vi "Calculate Tau Error.vi"(1 "tau":dbl, 2 "Dt":dbl, 3 "X":dbl[](array[numeric]), 4 "A":dbl, 8 "B":dbl) -> (7 "e_tau":dbl)   [LabVIEW 2019, in "Math Utilities.lvlib"]
doc: "Calculate the error in the fitted coefficient tau according to Halmer et al. [2004, Rev. Sci. Instr.]. The error will be the standard deviation of the fit (with N-3 degrees of freedom) multiplied by the sum of the square of the derivative of the exponential equation at each point in time."
uses:
  Math Utilities.lvlib
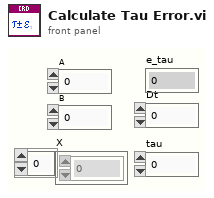
[diagram p1: front panel]
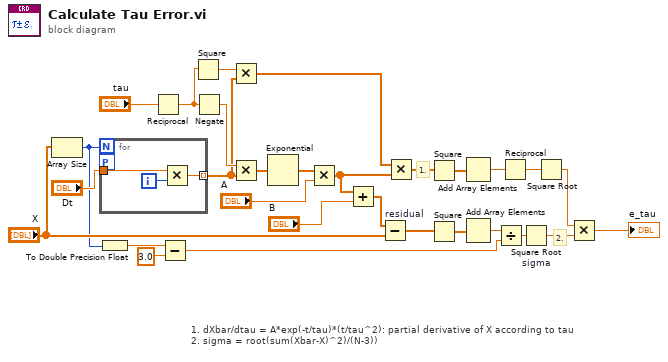
[diagram p0: block diagram]
diagram:
  # "2."
  # "1."
  # "1. dXbar/dtau = A*exp(-t/tau)*(t/tau^2): partial derivative of X according to tau\n2. sigma = root(sum(Xbar-X)^2)/(N-3))"
  n1 = Array Size(array="X") -> (size(s)=w11:i32)
  n2 = for {
    N: w11 -> [_]
    tunnel: "Dt" -> [w31]
    tunnel: [w30] -> w16 mode=indexing
    workers-P: _ -> [_]
    i -> [w32]
    n3 = Multiply(x=w31, y=w32) -> (x*y=w30:dbl)
  }
  n4 = To Double Precision Float(number=w11) -> (double precision float=w27:dbl)
  n5 = Reciprocal(x="tau") -> (1/x=w18:dbl)
  n6 = Subtract(x=w27, y=3.0) -> (x-y=w26:dbl)
  n7 = Square(x=w18) -> (x^2=w17:dbl)
  n8 = Negate(x=w18) -> (-x=w21:dbl)
  n9 = Multiply(x=w17, y=w16) -> (x*y=w15:dbl[])
  n10 = Multiply(x=w21, y=w16) -> (x*y=w22:dbl[])
  n11 = Exponential(1:w22) -> (0:w5:dbl[])
  n12 = Multiply(x=w5, y="A") -> (x*y=w1:dbl[])
  n13 = Add(x=w1, y="B") -> (x+y=w2:dbl[])
  n14 = Subtract "residual"(x=w2, y="X") -> (x-y=w10:dbl[])
  n15 = Multiply(x=w15, y=w1) -> (x*y=w14:dbl[])
  n16 = Square(x=w14) -> (x^2=w13:dbl[])
  n17 = Square(x=w10) -> (x^2=w23:dbl[])
  n18 = Add Array Elements(numeric array=w13) -> (sum=w7:dbl)
  n19 = Add Array Elements(numeric array=w23) -> (sum=w24:dbl)
  n20 = Divide ("sigma")(x=w24, y=w26) -> (x/y=w9:dbl)
  n21 = Reciprocal(x=w7) -> (1/x=w6:dbl)
  n22 = Square Root "sigma"(x=w9) -> (sqrt(x)=w8:dbl)
  n23 = Square Root(x=w6) -> (sqrt(x)=w12:dbl)
  n24 = Multiply(x=w12, y=w8) -> (x*y=→"e_tau":dbl)
